vi "ADIS16448 IMU Example.vi"() -> ()   [LabVIEW 2019]
uses:
  <vilib>/Utility/RT CPU Load.ctl
  ADIS16448Lib/Typedef/ADIS16448 Hardware Configuration.ctl
  <vilib>/Rock Robotics/WPI/SPI/WPI_SPIMode.ctl
  <vilib>/Rock Robotics/SystemInterfaces/DIO/FPGA_DIOChannel.ctl
  <vilib>/Rock Robotics/SystemInterfaces/spilib/spi_bus.ctl
  ADIS16448Lib/Typedef/ADIS16448 Data.ctl
  <vilib>/NI_Real-Time Target Support.lvlib
panel:
  out "ADIS16448 Value":T1
  out "IMU Detected?":bool
  in  "Calibration Time (sec)":u32=4
  in  "Hardware Config":T2={"SPI Clock Rate (Hz)"=1000000.0, "IMU SPI Mode (3)"=enum."Mode 3 (Clk Idle High,Sample on Trailing)", "IMU Reset Pin"=enum."DIO MXP 8", "IMU SPI Bus"=enum."SPI MXP", "IMU Data Ready Pin"=enum."DIO MXP 0", "Stall Config"={"Pow2BytesPerRead"=255, "StallTicks"=1000, "CsToSclkTicks"=5}, "IMU Status LED Pin"=enum."DIO MXP 9"}
  in  "Recalibrate?":bool
  in  "Reset?":bool
  out "Integrated Gyro Angle":T6(graph)
  out "Calibrated?":bool
  in  "Set Cal Time":bool
  out "CPU loads":T7[](array[typedef]) {"ISR (%)" format="%#.2f"; "Idle (%)" format="%#.2f"; "Background (%)" format="%#.2f"; "Normal (%)" format="%#.2f"; "Above Normal (%)" format="%#.2f"; "High (%)" format="%#.2g"; "Timed Structures (%)" format="%#.2g"; "Time Critical (%)" format="%#.2g"; "Total (%)" format="%#.2g"}
  in  "stop":bool
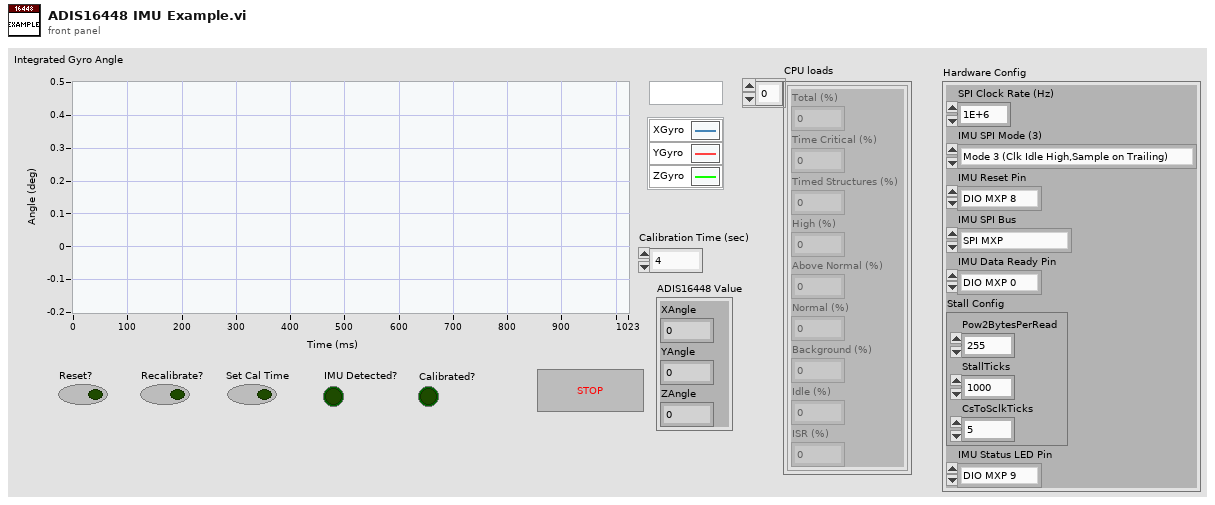
[diagram p1: front panel]
types:
  T1 = typedef "ADIS16448 Data.ctl" = cluster{"XAngle":dbl, "YAngle":dbl, "ZAngle":dbl}
  T2 = typedef "ADIS16448 Hardware Configuration.ctl" = cluster{"SPI Clock Rate (Hz)":dbl, "IMU SPI Mode (3)":T3, "IMU Reset Pin":T4, "IMU SPI Bus":T5, "IMU Data Ready Pin":T4, "Stall Config":cluster{"Pow2BytesPerRead":u8, "StallTicks":u16, "CsToSclkTicks":u8}, "IMU Status LED Pin":T4}
  T3 = typedef "WPI_SPIMode.ctl" = enum16{"Mode 0 (Clk Idle Low,Sample on Leading)", "Mode 1 (Clk Idle Low,Sample on Trailing)", "Mode 2 (Clk Idle High,Sample on Leading)", "Mode 3 (Clk Idle High,Sample on Trailing)"}
  T4 = typedef "FPGA_DIOChannel.ctl" = enum8{"DIO 0", "DIO 1", "DIO 2", "DIO 3", "DIO 4", "DIO 5", "DIO 6", "DIO 7", "DIO 8", "DIO 9", "DIO MXP 0", "DIO MXP 1", "DIO MXP 2", "DIO MXP 3", "DIO MXP 4", "DIO MXP 5", "DIO MXP 6", "DIO MXP 7", "DIO MXP 8", "DIO MXP 9", "DIO MXP 10", "DIO MXP 11", "DIO MXP 12", "DIO MXP 13", "DIO MXP 14", "DIO MXP 15", "SPI Port CS1", "SPI Port CS2", "SPI Port CS3", "SPI Port MISO", "SPI Port MOSI", "Invalid"}
  T5 = typedef "spi_bus.ctl" = enum16{"SPI On-Board, CS0", "SPI On-Board, CS1", "SPI On-Board, CS2", "SPI On-Board, CS3", "SPI MXP", "Invalid"}
  T6 = cluster{"XAngle":dbl, "YAngle":dbl, "ZAngle":dbl}
  T7 = typedef "NI_Real-Time Target Support.lvlib/RT CPU Load.ctl" = cluster{"Total (%)":dbl, "Time Critical (%)":dbl, "Timed Structures (%)":dbl, "High (%)":dbl, "Above Normal (%)":dbl, "Normal (%)":dbl, "Background (%)":dbl, "Idle (%)":dbl, "ISR (%)":dbl}
  T8 = typedef "ADIS16448 Device Reference.ctl" = cluster{"DevStatus":errorcluster, "Hardware Config":T2, "Calibration Complete":refnum<notifier>, "Status FIFO":refnum<k33>, "Last Value Reference":refnum<data-value>, "Sychronous Process VI":T9, "Cmd FIFO":refnum<k33>, "Source":T10, "Data FIFO":refnum<k33>, "IMU Status LED Pin":T4, "Calibration Time":u32}
  T9 = typedef "ADIS16448 Process.ctl" = refnum<vi>
  T10 = typedef "FPGA_CounterEncoderSourceConvertionLVSourceType.ctl" = cluster{"DevStatus":errorcluster, "AnalogTriggerMode?":bool, "DigitalMode":cluster{"DIO Channel":T11}, "AnalogTriggerMode":cluster{"AnalogTriggerIndex":T12, "OutputType":T13}}
  T11 = typedef "FPGA_DIODigitalSourceChannel.ctl" = enum8{"DIO 0", "DIO 1", "DIO 2", "DIO 3", "DIO 4", "DIO 5", "DIO 6", "DIO 7", "DIO 8", "DIO 9", "DIO MXP 0", "DIO MXP 1", "DIO MXP 2", "DIO MXP 3", "DIO MXP 4", "DIO MXP 5", "DIO MXP 6", "DIO MXP 7", "DIO MXP 8", "DIO MXP 9", "DIO MXP 10", "DIO MXP 11", "DIO MXP 12", "DIO MXP 13", "DIO MXP 14", "DIO MXP 15", "SPI Port CS1", "SPI Port CS2", "SPI Port CS3", "SPI Port MISO", "SPI Port MOSI", "Disabled"}
  T12 = typedef "FPGA_AnalogTriggerIndex.ctl" = enum8{"Trig 0", "Trig 1", "Trig 2", "Trig 3", "Trig 4", "Trig 5", "Trig 6", "Trig 7", "Invalid"}
  T13 = typedef "FPGA_AnalogTriggerOutType.ctl" = enum16{"InWindow", "TriggerState", "Rising", "Falling"}
  T14 = typedef "ADIS16448 Status.ctl" = cluster{"Calibrated?":bool, "IMU Detected?":bool}
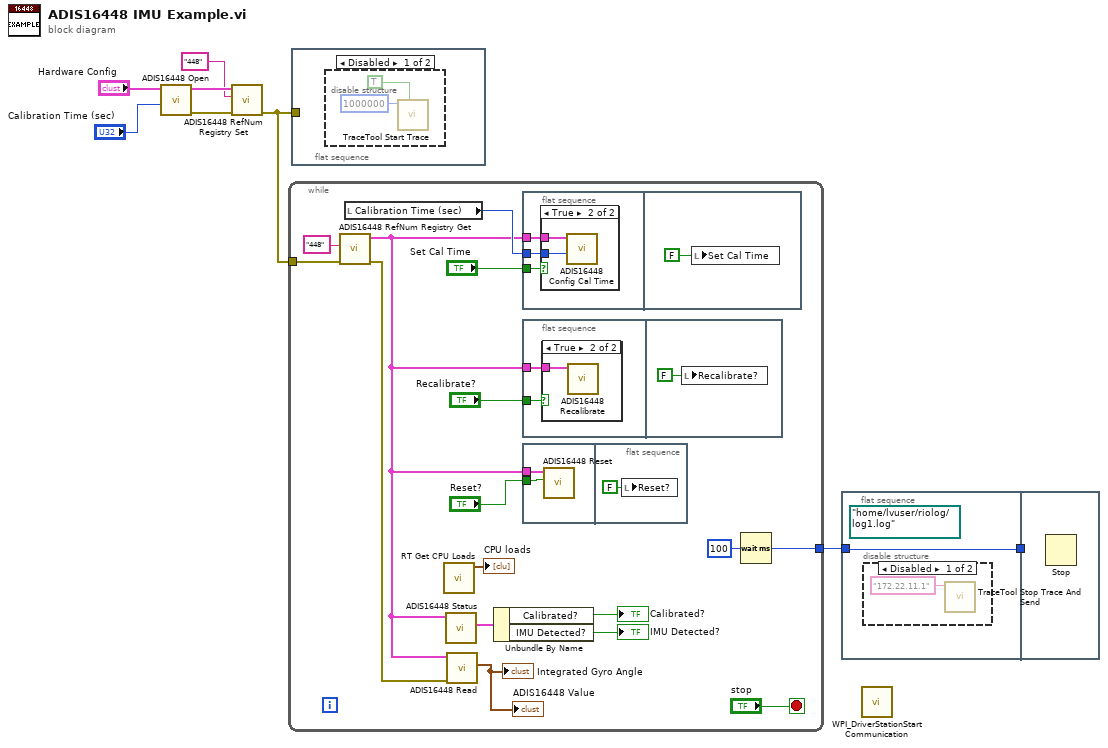
[diagram p0: block diagram]
diagram:
  n1 = call "ADIS16448 Open.vi"("Initial Calibration Time (sec)"="Calibration Time (sec)", "Hardware Config"="Hardware Config") -> ("error out"=w4:errorcluster, "ADIS16448DevRef"=w3:T8)  [unwired: 8 in]
  n2 = call "ADIS16448 RefNum Registry Set.vi"("error in (no error)"=w4, "refnum name"="448", "ADIS16448DevRef"=w3) -> ("error out"=w1:errorcluster)  [unwired: 7 in, 1 out]
  n3 = while {
    tunnel: [w21] -> w8
    tunnel: w1 -> [w10]
    stop <- "stop" stop-if-true
    n4 = call "ADIS16448 RefNum Registry Get.vi"("error in (no error)"=w10, "refnum name"="448") -> ("error out"=w9:errorcluster, "ADIS16448DevRef Out"=w12:T8)  [unwired: 8 in]
    n5 = local read "Calibration Time (sec)"() -> (w14:u32)
    n6 = call <vilib>:"RT Get CPU Loads.vi"() -> ("CPU loads"=→"CPU loads":T7[])  [unwired: 10 in, 1 out]
    n7 = call "ADIS16448 Status.vi"("ADIS16448DevRef"=w12) -> ("ADIS16448 Status"=w19:T14)  [unwired: 8 in, 2 out]
    n8 = call "ADIS16448 Read.vi"("error in (no error)"=w9, "ADIS16448DevRef"=w12) -> ("ADIS16448 Value"=→"Integrated Gyro Angle" →"ADIS16448 Value":T1)  [unwired: 6 in, 3 out]
    n9 = Unbundle By Name(w19) -> ("Calibrated?"=→"Calibrated?":bool, "IMU Detected?"=→"IMU Detected?":bool)
    n10 = flat-sequence {
      tunnel: "Set Cal Time" -> [w27]
      tunnel: w14 -> [w26]
      tunnel: w12 -> [w25]
      frame #0 {
        n11 = case shown="True" w27 {
          tunnel: w26 -> [_ w29]
          tunnel: w25 -> [_ w28]
          frame False {
          }
          frame True {
            n12 = call "ADIS16448 Config Cal Time.vi"("Data"=w29, "ADIS16448DevRef in"=w28) -> ()  [unwired: 8 in, 2 out]
          }
        }
      }
      frame #1 {
        n13 = local write "Set Cal Time"(FALSE ("Ready?")) -> ()
      }
    }
    n14 = flat-sequence {
      tunnel: "Recalibrate?" -> [w32]
      tunnel: w12 -> [w31]
      frame #0 {
        n15 = case shown="True" w32 {
          tunnel: w31 -> [_ w33]
          frame False {
          }
          frame True {
            n16 = call "ADIS16448 Recalibrate.vi"("ADIS16448DevRef in"=w33) -> ()  [unwired: 9 in, 2 out]
          }
        }
      }
      frame #1 {
        n17 = local write "Recalibrate?"(FALSE ("Recalibrate?")) -> ()
      }
    }
    n18 = flat-sequence {
      tunnel: "Reset?" -> [w36]
      tunnel: w12 -> [w35]
      frame #0 {
        n19 = call "ADIS16448 Reset.vi"("Reset?"=w36, "ADIS16448DevRef"=w35) -> ()  [unwired: 8 in, 2 out]
      }
      frame #1 {
        n20 = local write "Reset?"(FALSE ("Reset?")) -> ()
      }
    }
    n21 = Wait (ms)(milliseconds to wait=u32 100) -> (millisecond timer value=w21:u32)
  }
  n22 = flat-sequence {
    tunnel: w1 -> [_]
    frame #0 {
      n23 = disable-structure shown="Disabled" {
        frame Disabled {
          n24 = call <vilib>:"TraceTool Start Trace.vi"("Detailed Tracing? (F)"=TRUE, "Buffer Size (250000 bytes)"=1000000) -> ()  [unwired: 8 in, 2 out]
        }
        frame Enabled {
        }
      }
    }
  }
  n25 = flat-sequence {
    tunnel: w8 -> [w40]
    tunnel: [w40] -> w7
    tunnel: w7 -> [_]
    frame #0 {
      (unwired) path "/home/lvuser/riolog/log1.log" ("Path to Trace Log")
      n26 = disable-structure shown="Disabled" {
        frame Disabled {
          n27 = call <vilib>:"TraceTool Stop Trace And Send.vi"("Trace Host Network Address"="172.22.11.1") -> ()  [unwired: 10 in, 1 out]
        }
        frame Enabled {
        }
      }
    }
    frame #1 {
      n28 = Stop() -> ()  [unwired: 1 in]
    }
  }
  n29 = call <vilib>:"WPI_DriverStationStart Communication.vi"() -> ()  [unwired: 12 in]
